vi "PCI1220U双轴初始化.vi"(5 "Device Type":u16(ring) items=["PCI-1220 (M0)"]) -> (1 "输出轴AxisHandle OUT":u32, 2 "输入轴AxisHandle OUT":u32, 3 "DeviceHandle":u32, 4 "Device Type 2":u16(ring) items=["PCI-1220 (M0)"])   [LabVIEW 2013]
panel:
  out "ReturnValue 8":u32
  out "ReturnValue 7":u32
  out "ReturnValue 6":u32
  out "ReturnValue 5":u32
  out "ReturnValue 4":u32
  out "ReturnValue 3":u32
  out "ReturnValue 2":u32
  out "ReturnValue":u32
  out "DevAxesCount":u32
  out "AxisOpened":bool
  out "DeviceNum List":u32[](array[numeric])
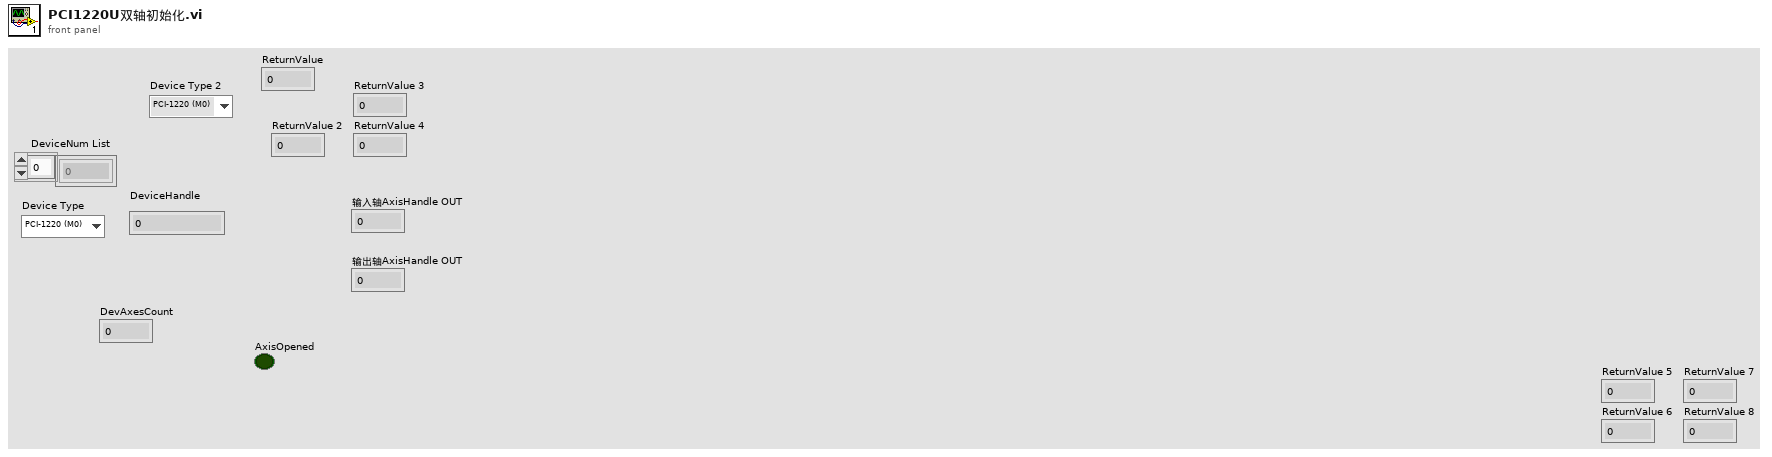
[diagram p1: front panel]
types:
  T1 = cluster{"DeviceNum":u32, "U*8 Array":cluster{"U*8 Array[0]":u8, "U*8 Array[1]":u8, "U*8 Array[2]":u8, "U*8 Array[3]":u8, "U*8 Array[4]":u8, "U*8 Array[5]":u8, "U*8 Array[6]":u8, "U*8 Array[7]":u8, "U*8 Array[8]":u8, "U*8 Array[9]":u8, "U*8 Array[10]":u8, "U*8 Array[11]":u8, "U*8 Array[12]":u8, "U*8 Array[13]":u8, "U*8 Array[14]":u8, "U*8 Array[15]":u8, "U*8 Array[16]":u8, "U*8 Array[17]":u8, "U*8 Array[18]":u8, "U*8 Array[19]":u8, "U*8 Array[20]":u8, "U*8 Array[21]":u8, "U*8 Array[22]":u8, "U*8 Array[23]":u8, "U*8 Array[24]":u8, "U*8 Array[25]":u8, "U*8 Array[26]":u8, "U*8 Array[27]":u8, "U*8 Array[28]":u8, "U*8 Array[29]":u8, "U*8 Array[30]":u8, "U*8 Array[31]":u8, "U*8 Array[32]":u8, "U*8 Array[33]":u8, "U*8 Array[34]":u8, "U*8 Array[35]":u8, "U*8 Array[36]":u8, "U*8 Array[37]":u8, "U*8 Array[38]":u8, "U*8 Array[39]":u8, "U*8 Array[40]":u8, "U*8 Array[41]":u8, "U*8 Array[42]":u8, "U*8 Array[43]":u8, "U*8 Array[44]":u8, "U*8 Array[45]":u8, "U*8 Array[46]":u8, "U*8 Array[47]":u8, "U*8 Array[48]":u8, "U*8 Array[49]":u8}, "NumOfSubDevice":i16}[]
  T2 = cluster{"U*8 Array[0]":u8, "U*8 Array[1]":u8, "U*8 Array[2]":u8, "U*8 Array[3]":u8, "U*8 Array[4]":u8, "U*8 Array[5]":u8, "U*8 Array[6]":u8, "U*8 Array[7]":u8, "U*8 Array[8]":u8, "U*8 Array[9]":u8, "U*8 Array[10]":u8, "U*8 Array[11]":u8, "U*8 Array[12]":u8, "U*8 Array[13]":u8, "U*8 Array[14]":u8, "U*8 Array[15]":u8, "U*8 Array[16]":u8, "U*8 Array[17]":u8, "U*8 Array[18]":u8, "U*8 Array[19]":u8, "U*8 Array[20]":u8, "U*8 Array[21]":u8, "U*8 Array[22]":u8, "U*8 Array[23]":u8, "U*8 Array[24]":u8, "U*8 Array[25]":u8, "U*8 Array[26]":u8, "U*8 Array[27]":u8, "U*8 Array[28]":u8, "U*8 Array[29]":u8, "U*8 Array[30]":u8, "U*8 Array[31]":u8, "U*8 Array[32]":u8, "U*8 Array[33]":u8, "U*8 Array[34]":u8, "U*8 Array[35]":u8, "U*8 Array[36]":u8, "U*8 Array[37]":u8, "U*8 Array[38]":u8, "U*8 Array[39]":u8, "U*8 Array[40]":u8, "U*8 Array[41]":u8, "U*8 Array[42]":u8, "U*8 Array[43]":u8, "U*8 Array[44]":u8, "U*8 Array[45]":u8, "U*8 Array[46]":u8, "U*8 Array[47]":u8, "U*8 Array[48]":u8, "U*8 Array[49]":u8}
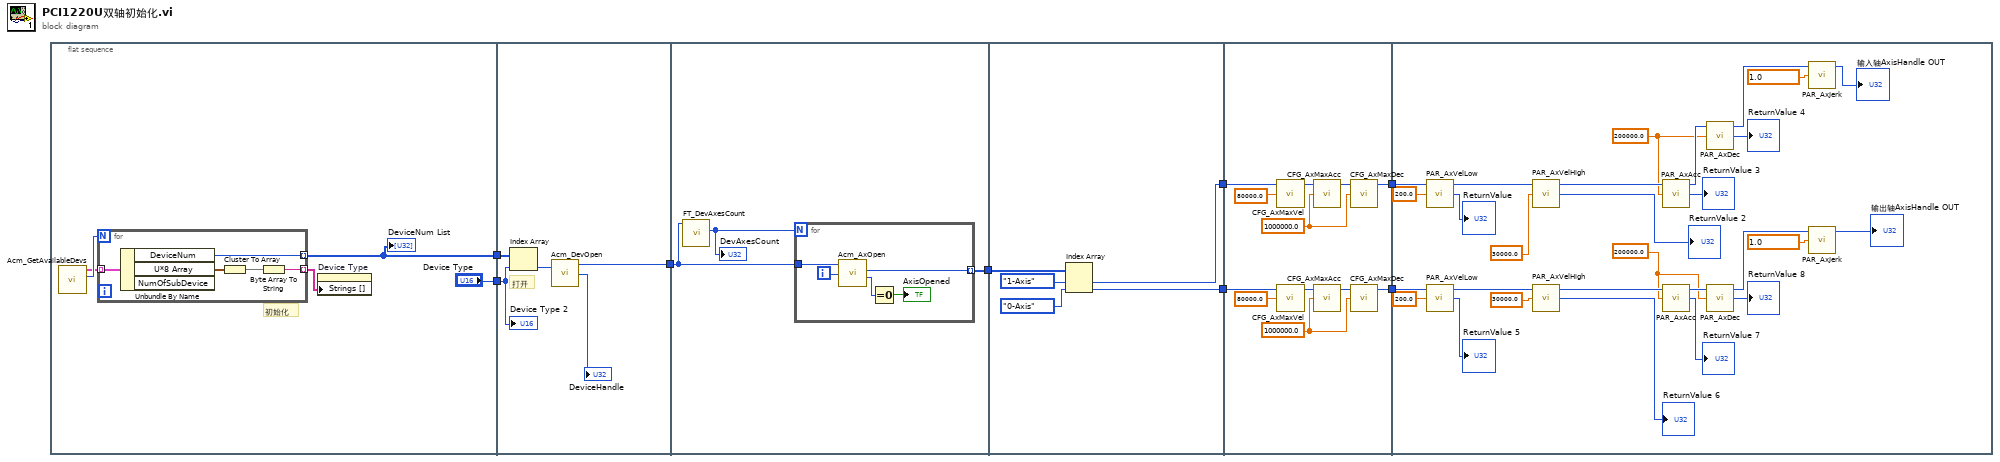
[diagram p0: block diagram]
diagram:
  n1 = flat-sequence {
    tunnel: [w10] -> w8
    tunnel: ["Device Type"] -> w7
    tunnel: w8 -> [w23]
    tunnel: w7 -> [w19]
    tunnel: [w21] -> w6
    tunnel: w6 -> [w25]
    tunnel: [w24] -> w5
    tunnel: w5 -> [w36]
    tunnel: [w34] -> w4
    tunnel: [w32] -> w2
    tunnel: w4 -> [w48]
    tunnel: [w47] -> w3
    tunnel: w2 -> [w46]
    tunnel: [w45] -> w1
    tunnel: w3 -> [w76]
    tunnel: w1 -> [w75]
    frame #0 {
      # "初始化"
      n2 = call <userlib>:"Acm_GetAvailableDevs.vi"() -> ("OutEntries"=w13:u32, "DeviceList"=w12:T1)  [unwired: 1 in, 2 out]
      n3 = for {
        N: w13 -> [_]
        tunnel: w12 -> [w18] mode=indexing
        tunnel: [w15] -> w10 mode=indexing
        tunnel: [w14] -> w11 mode=indexing
        n4 = Unbundle By Name(w18) -> ("DeviceNum"=w15:u32, "U*8 Array"=w17:T2)  [unwired: 1 out]
        n5 = Cluster To Array(cluster=w17) -> (array=w16:u8[])
        n6 = Byte Array To String(unsigned byte array=w16) -> (string=w14:string)
      }
      "DeviceNum List" <- w10
      n7 = property on="Device Type" class="Ring (严格)"("Strings []"=w11) -> ()  [unwired: 2 in, 2 out]
    }
    frame #1 {
      # "打开"
      n8 = Index Array(array=w23, index=w19) -> (element=w22:u32)
      n9 = call <userlib>:"Acm_DevOpen.vi"("DeviceNumber"=w22) -> ("ReturnValue"=→"DeviceHandle":u32, "DeviceHandle"=w21:u32)  [unwired: 1 in, 1 out]
      "Device Type 2" <- w19
    }
    frame #2 {
      n10 = call <userlib>:"FT_DevAxesCount.vi"("Handle"=w25) -> ("DevAxesCount"=w26:u32)  [unwired: 1 in, 6 out]
      "DevAxesCount" <- w26
      n11 = for {
        N: w26 -> [_]
        tunnel: w25 -> [w31]
        tunnel: [w27] -> w24 mode=indexing
        i -> [w30]
        n12 = call <userlib>:"Acm_AxOpen.vi"("PhyAxis"=w30, "DeviceHandle"=w31) -> ("ReturnValue"=w29:u32, "AxisHandle"=w27:u32)  [unwired: 1 in, 2 out]
        n13 = Equal To 0?(x=w29) -> (x = 0?=→"AxisOpened":bool)
      }
    }
    frame #3 {
      n14 = Index Array(array=w36, index #1=enum32{"0-Axis", "1-Axis", "2-Axis", "3-Axis"}."1-Axis" ("Operate Axis"), index #2=enum32{"0-Axis", "1-Axis", "2-Axis", "3-Axis"}."0-Axis" ("Operate Axis")) -> (element #1=w34:u32, element #2=w32:u32)
    }
    frame #4 {
      w40 = 1000000.0 ("CFG_AxMaxAcc")
      w44 = 1000000.0 ("CFG_AxMaxAcc")
      n15 = call <userlib>:"CFG_AxMaxVel.vi"("CFG_AxMaxVel"=80000.0, "Handle"=w48) -> ("Handle 2"=w42:u32)  [unwired: 1 in, 2 out]
      n16 = call <userlib>:"CFG_AxMaxVel.vi"("CFG_AxMaxVel"=80000.0, "Handle"=w46) -> ("Handle 2"=w38:u32)  [unwired: 1 in, 2 out]
      n17 = call <userlib>:"CFG_AxMaxAcc.vi"("CFG_AxMaxAcc"=w44, "Handle"=w42) -> ("Handle 2"=w43:u32)  [unwired: 1 in, 2 out]
      n18 = call <userlib>:"CFG_AxMaxAcc.vi"("CFG_AxMaxAcc"=w40, "Handle"=w38) -> ("Handle 2"=w39:u32)  [unwired: 1 in, 2 out]
      n19 = call <userlib>:"CFG_AxMaxDec.vi"("CFG_AxMaxDec"=w44, "Handle"=w43) -> ("Handle 2"=w47:u32)  [unwired: 1 in, 2 out]
      n20 = call <userlib>:"CFG_AxMaxDec.vi"("CFG_AxMaxDec"=w40, "Handle"=w39) -> ("Handle 2"=w45:u32)  [unwired: 1 in, 2 out]
    }
    frame #5 {
      w55 = 1.0 items=["T-curve", "S-curve"] ("PAR_AxJerk")
      w56 = 200000.0 ("PAR_AxAcc")
      w67 = 1.0 items=["T-curve", "S-curve"] ("PAR_AxJerk")
      w68 = 200000.0 ("PAR_AxAcc")
      n21 = call <userlib>:"PAR_AxVelLow.vi"("PAR_AxVelLow"=200.0, "Handle"=w76) -> ("ReturnValue"=→"ReturnValue":u32, "Handle 2"=w74:u32)  [unwired: 1 in, 1 out]
      n22 = call <userlib>:"PAR_AxVelLow.vi"("PAR_AxVelLow"=200.0, "Handle"=w75) -> ("ReturnValue"=→"ReturnValue 5":u32, "Handle 2"=w62:u32)  [unwired: 1 in, 1 out]
      n23 = call <userlib>:"PAR_AxVelHigh.vi"("PAR_AxVelHigh"=30000.0, "Handle"=w74) -> ("ReturnValue"=→"ReturnValue 2":u32, "Handle 2"=w73:u32)  [unwired: 1 in, 1 out]
      n24 = call <userlib>:"PAR_AxVelHigh.vi"("PAR_AxVelHigh"=30000.0, "Handle"=w62) -> ("ReturnValue"=→"ReturnValue 6":u32, "Handle 2"=w61:u32)  [unwired: 1 in, 1 out]
      n25 = call <userlib>:"PAR_AxAcc.vi"("PAR_AxAcc"=w68, "Handle"=w73) -> ("ReturnValue"=→"ReturnValue 3":u32, "Handle 2"=w72:u32)  [unwired: 1 in, 1 out]
      n26 = call <userlib>:"PAR_AxAcc.vi"("PAR_AxAcc"=w56, "Handle"=w61) -> ("ReturnValue"=→"ReturnValue 7":u32, "Handle 2"=w60:u32)  [unwired: 1 in, 1 out]
      n27 = call <userlib>:"PAR_AxDec.vi"("PAR_AxDec"=w68, "Handle"=w72) -> ("ReturnValue"=→"ReturnValue 4":u32, "Handle 2"=w71:u32)  [unwired: 1 in, 1 out]
      n28 = call <userlib>:"PAR_AxDec.vi"("PAR_AxDec"=w56, "Handle"=w60) -> ("ReturnValue"=→"ReturnValue 8":u32, "Handle 2"=w59:u32)  [unwired: 1 in, 1 out]
      n29 = call <userlib>:"PAR_AxJerk.vi"("PAR_AxJerk"=w67, "Handle"=w71) -> ("Handle 2"=→"输入轴AxisHandle OUT":u32)  [unwired: 1 in, 2 out]
      n30 = call <userlib>:"PAR_AxJerk.vi"("PAR_AxJerk"=w55, "Handle"=w59) -> ("Handle 2"=→"输出轴AxisHandle OUT":u32)  [unwired: 1 in, 2 out]
    }
  }
